vi "Actuate.vi"(0 "Single Cylinder Actuator in":refnum<class "Single Cylinder Actuator.lvclass">, 5 "FC1 ILC in":refnum<class "ILC.lvclass">, 7 "FC2 ILC in":refnum<class "ILC.lvclass">, 9 "Actuate Arguments":T3 {"FC2 Measured Value" format="%.3f"; "Lateral Demand" format="%.3f"; "FC1 Measured Value" format="%.3f"; "Axial Demand" format="%.3f"}, 11 "error in (no error)":errorcluster) -> (4 "Single Cylinder Actuator out":refnum<class "Single Cylinder Actuator.lvclass">, 6 "FC1 ILC out":refnum<class "ILC.lvclass">, 8 "FC2 ILC out":refnum<class "ILC.lvclass">, 10 "Actuate Results":T1 {"FC2 Demand" format="%.3f"; "FC1 Demand" format="%.3f"}, 15 "error out":errorcluster)   [LabVIEW 2015, in "Single Cylinder Actuator.lvclass"]
uses:
  Single Cylinder Actuator.lvclass
  <userlib>/Common/ILC/ILC/ILC.lvclass
  Typedefs/Actuate Arguments.ctl
  Typedefs/Actuate Results.ctl
  Typedefs/Cylinder Results.ctl
  Single Cylinder Actuator.lvclass/Single Cylinder Actuator.ctl
  Actuator Cylinder/Actuator Cylinder/Actuator Cylinder.lvclass
  Typedefs/FAMT Typedefs.lvlib
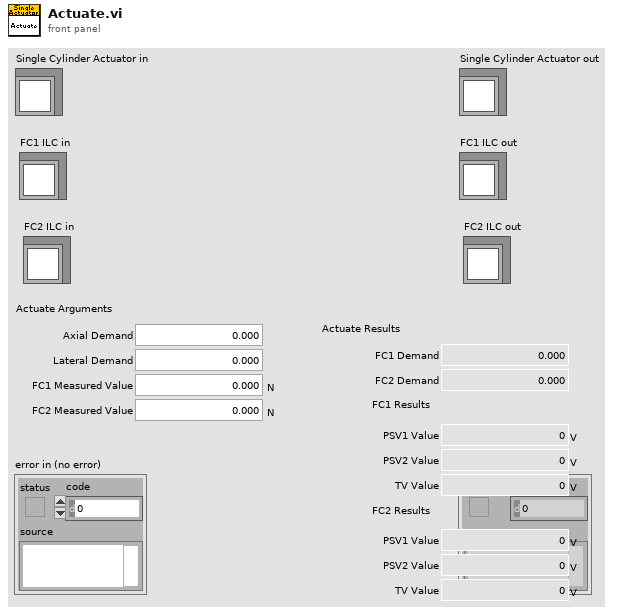
[diagram p1: front panel]
types:
  T1 = typedef "FAMT Typedefs.lvlib/Actuate Results.ctl" = cluster{"FC1 Demand":dbl, "FC2 Demand":dbl, "FC1 Results":T2, "FC2 Results":T2}
  T2 = typedef "FAMT Typedefs.lvlib/Cylinder Results.ctl" = cluster{"PSV1 Value":dbl[unit], "PSV2 Value":dbl[unit], "TV Value":dbl[unit]}
  T3 = typedef "FAMT Typedefs.lvlib/Actuate Arguments.ctl" = cluster{"Axial Demand":dbl, "Lateral Demand":dbl, "FC1 Measured Value":dbl[unit], "FC2 Measured Value":dbl[unit]}
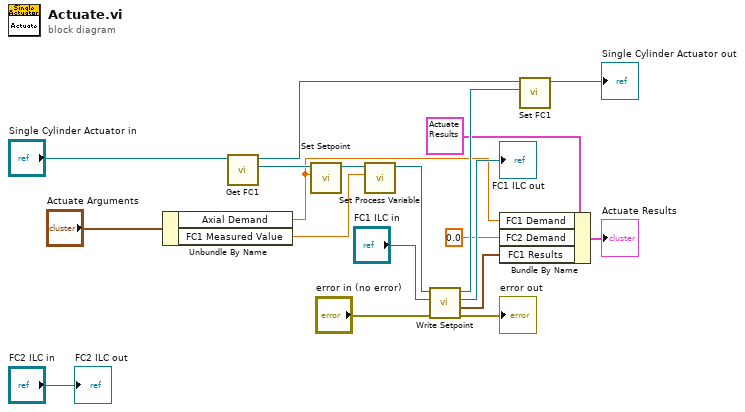
[diagram p0: block diagram]
diagram:
  n1 = Unbundle By Name("Actuate Arguments") -> ("Axial Demand"=w3:dbl, "FC1 Measured Value"=w16:dbl[unit])
  n2 = call "Get FC1.vi"("SingleCylinderActuator in"="Single Cylinder Actuator in") -> ("FC1"=w18:refnum<class "Actuator Cylinder.lvclass">, "SingleCylinderActuator out"=w8:refnum<class "Single Cylinder Actuator.lvclass">)  [unwired: 9 in]
  n3 = call-dynamic "Set Setpoint.vi"("Setpoint"=w3, "Actuator Cylinder in"=w18) -> ("Actuator Cylinder out"=w15:refnum<class "Actuator Cylinder.lvclass">)  [unwired: 9 in]
  n4 = call-dynamic "Set Process Variable.vi"("Process Variable"=w16, "Actuator Cylinder in"=w15) -> ("Actuator Cylinder out"=w10:refnum<class "Actuator Cylinder.lvclass">)  [unwired: 9 in]
  n5 = call-dynamic "Write Setpoint.vi"("error in (no error)"="error in (no error)", "ILC in"="FC1 ILC in", "Actuator Cylinder in"=w10) -> ("error out"=→"error out":errorcluster, "Cylinder Results"=w1:T2, "ILC out"=→"FC1 ILC out":refnum<class "ILC.lvclass">, "Actuator Cylinder out"=w9:refnum<class "Actuator Cylinder.lvclass">)  [unwired: 5 in]
  n6 = Bundle By Name(cluster=T1 {"FC1 Demand"=0.0, "FC2 Demand"=0.0, "FC1 Results"={"PSV1 Value"=0.0, "PSV2 Value"=0.0, "TV Value"=0.0}, "FC2 Results"={"PSV1 Value"=0.0, "PSV2 Value"=0.0, "TV Value"=0.0}} ("Actuate Results"), "FC1 Demand"=w3, "FC2 Demand"=0.0, "FC1 Results"=w1) -> (→"Actuate Results":T1)
  n7 = call "Set FC1.vi"("FC1"=w9, "SingleCylinderActuator in"=w8) -> ("SingleCylinderActuator out"=→"Single Cylinder Actuator out":refnum<class "Single Cylinder Actuator.lvclass">)  [unwired: 9 in]
  "FC2 ILC out" <- "FC2 ILC in"
